vi "gf3.vi"(4 "Waveform":waveform(dbl), 6 "T":dbl=10.0 format="%#_3p") -> (1 "Waveform 2":waveform(dbl), 2 "T":dbl)   [LabVIEW 2010]
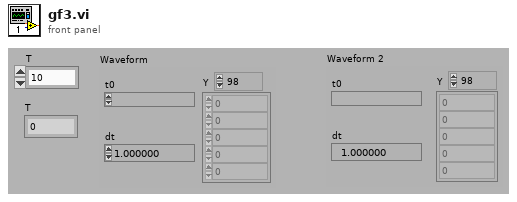
[diagram p1: front panel]
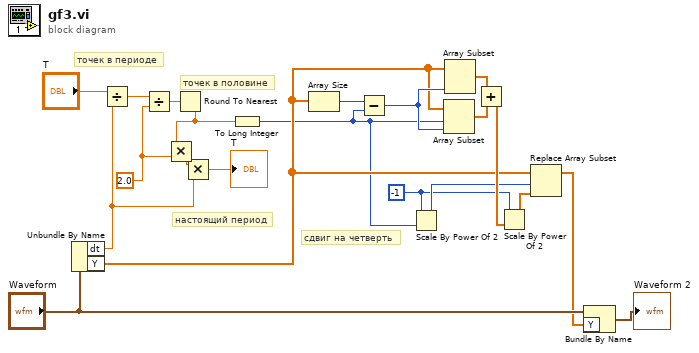
[diagram p0: block diagram]
diagram:
  w1 = -1 ("index")
  w2 = 2.0 ("n")
  # "сдвиг на четверть"
  # "настоящий период"
  # "точек в половине"
  # "точек в периоде"
  n1 = Unbundle By Name("Waveform") -> ("dt"=w3:dbl, "Y"=w6:dbl[])
  n2 = Divide(x="T", y=w3) -> (x/y=w17:dbl)
  n3 = Divide(x=w17, y=w2) -> (x/y=w18:dbl)
  n4 = Round To Nearest(number=w18) -> (nearest integer value=w10:dbl)
  n5 = Multiply(x=w10, y=w2) -> (x*y=w12:dbl)
  n6 = Multiply(x=w12, y=w3) -> (x*y=→"T":dbl)
  n7 = To Long Integer(number=w10) -> (32bit integer=w5:i32)
  n8 = Array Size(array=w6) -> (size(s)=w13:i32)
  n9 = Subtract(x=w13, y=w5) -> (x-y=w7:i32)
  n10 = Scale By Power Of 2(n=w1, x=w5) -> (x*2^n=w4:i32)
  n11 = Array Subset(array=w6, index=w5, length=w7) -> (w15:dbl[])
  n12 = Array Subset(array=w6, length=w7) -> (w16:dbl[])  [unwired: 1 in]
  n13 = Add(x=w16, y=w15) -> (x+y=w14:dbl[])
  n14 = Scale By Power Of 2(n=w1, x=w14) -> (x*2^n=w9:dbl[])
  n15 = Replace Array Subset(array=w6, new element=w9, index=w4) -> (w8:dbl[])
  n16 = Bundle By Name(cluster="Waveform", "Y"=w8) -> (→"Waveform 2":waveform(dbl))
